vi "VIE.Module.Queued Message Handler.QueuedMessageHandler_setModifiedData(NoError).vi"(0 "reference":T1, 2 "data":T2) -> (14 "duplicate reference":T1, 19 "error out":errorcluster)   [LabVIEW 2010, in "VIE.Module.Queued Message Handler.QueuedMessageHandler.dqGOOPClass.lvlib"]
doc: "This VI writes the data of the dqGOOP object and unlocks it for write access. There is no Error In cluster so the original data doesn't need to be passed in. This provides a performance improvement for objects with a large data store, when the write method can not generate an internal error."
uses:
  VIE.Module.Queued Message Handler.QueuedMessageHandler.dqGOOPClass.lvlib
  VIE.Module.Queued Message Handler.dqClass_ObjectReference.ctl
  VIE.Module.Queued Message Handler.dqClass_ObjectData.ctl
panel:
  in  "queue (default)":refnum<queue>
  # "Copyright (C) 2004 DataAct Incorporated"
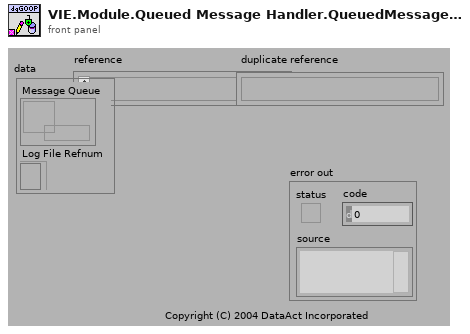
[diagram p1: front panel]
types:
  T1 = typedef "VIE.Module.Queued Message Handler.QueuedMessageHandler.dqGOOPClass.lvlib/VIE.Module.Queued Message Handler.dqClass_ObjectReference.ctl" = refnum<k1>
  T2 = typedef "VIE.Module.Queued Message Handler.QueuedMessageHandler.dqGOOPClass.lvlib/VIE.Module.Queued Message Handler.dqClass_ObjectData.ctl" = cluster{"Message Queue":refnum<queue>, "Log File Refnum":refnum<file>}
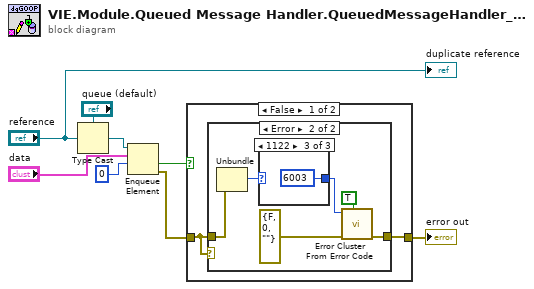
[diagram p0: block diagram]
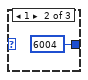
[diagram p4: hidden frame]
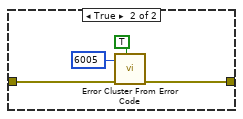
[diagram p5: hidden frame]
diagram:
  n1 = Type Cast(type="queue (default)", x="reference") -> (*(type *) &x=w1:refnum<queue>)
  n2 = Enqueue Element(queue=w1, element="data", timeout in ms (-1)=0 ("timeout in ms (0)")) -> (timed out?=w6:bool, error out=w8:errorcluster)  [unwired: 1 in, 1 out]
  n3 = case shown="False" w6 {
    tunnel: w8 -> [w10 w22]
    tunnel: [w9 w21] -> w7
    frame False {
      n4 = case shown="Error" w10 {
        tunnel: [w11 w12] -> w9
        tunnel: w10 -> [w11 w17]
        frame No Error {
        }
        frame Error {
          n5 = Unbundle(w17) -> ("code"=w16:i32)  [unwired: 2 out]
          n6 = case shown="1122" w16 {
            selector: w16 -> [w18 _ _]
            tunnel: [w18 6004 ("code") 6003 ("code")] -> w14
            frame Default {
            }
            frame 1 {
            }
            frame 1122 {
            }
          }
          n7 = call <vilib>:"Error Cluster From Error Code.vi"("show call chain? (False)"=TRUE, "error in (no error)"=errorcluster {"status"=FALSE, "code"=0, "source"=""} ("error out"), "error code (0)"=w14) -> ("error out"=w12:errorcluster)  [unwired: 6 in]
        }
      }
    }
    frame True {
      n8 = call <vilib>:"Error Cluster From Error Code.vi"("show call chain? (False)"=TRUE, "error in (no error)"=w22, "error code (0)"=6005 ("code")) -> ("error out"=w21:errorcluster)  [unwired: 6 in]
    }
  }
  "error out" <- w7
  "duplicate reference" <- "reference"
